vi "PhotonPipelineResult_HasTargets.vi"(11 "PhotonPipelineResult_REF":T1) -> (3 "HasTargets":bool)   [LabVIEW 2019, in "PhotonVisionLib.lvlib"]
doc: "Returns whether the pipeline has targets.\n\nInputs:\n - PipelineResult -- Parsed PipelineResult cluster.\n\nOutputs:\n - HasTargets -- Whether the pipeline has targets."
uses:
  PhotonVisionLib.lvlib
  TypeDef/PhotonPipelineResultType.ctl
  TypeDef/PhotonTrackedTargetType.ctl
  TypeDef/TargetCornerType.ctl
  <vilib>/Rock Robotics/WPI/ThirdParty/JAS_Junk/TrajLib/TypeDef/TRANSFORM3D.ctl
  <vilib>/Rock Robotics/WPI/ThirdParty/JAS_Junk/TrajLib/TypeDef/TRANSLATION3D.ctl
  <vilib>/Rock Robotics/WPI/ThirdParty/JAS_Junk/TrajLib/TypeDef/ROTATION3D.ctl
  <vilib>/Rock Robotics/WPI/ThirdParty/JAS_Junk/TrajLib/TypeDef/QUATERNION.ctl
  TypeDef/PhotonMultiTargetPNPResultType.ctl
  TypeDef/PhotonPNPResultType.ctl
  <vilib>/Rock Robotics/WPI/ThirdParty/JAS_Junk/TrajLib/Trajectory_Library.lvlib
  Ref/PhotonPipelineResult_REF.ctl
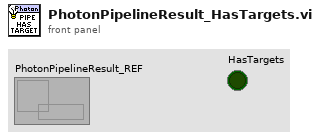
[diagram p1: front panel]
types:
  T1 = typedef "PhotonVisionLib.lvlib/PhotonPipelineResult_REF.ctl" = refnum<data-value>
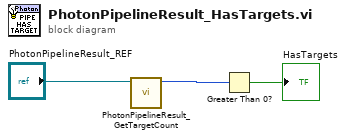
[diagram p0: block diagram]
diagram:
  n1 = call "PhotonPipelineResult_GetTargetCount.vi"("PhotonPipelineResult_REF"="PhotonPipelineResult_REF") -> ("TargetCount"=w1:i32)  [unwired: 10 in]
  n2 = Greater Than 0?(x=w1) -> (x > 0?=→"HasTargets":bool)
